vi "GDSString_CapsAndRemoveSpaces.vi"(10 "String":string) -> (2 "concatenated string":string)   [LabVIEW 2020]
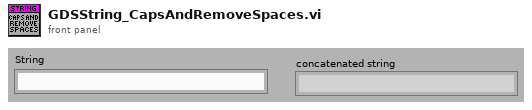
[diagram p1: front panel]
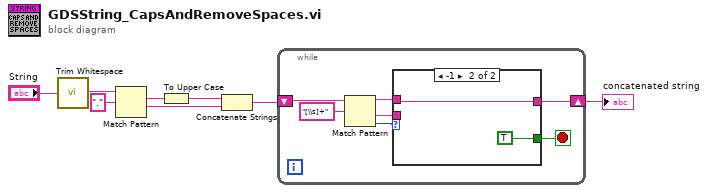
[diagram p0: block diagram]
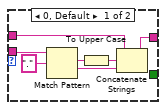
[diagram p2: hidden frame]
diagram:
  n1 = call <vilib>:"Trim Whitespace.vi"("string"="String") -> ("trimmed string"=w7:string)  [unwired: 1 in]
  n2 = Match Pattern(string=w7, regular expression=".") -> (match substring=w5:string, after substring=w3:string)  [unwired: 1 in, 2 out]
  n3 = To Upper Case(1:w5) -> (0:w4:string)
  n4 = Concatenate Strings(w4, w3) -> (w2:string)
  n5 = while {
    shift-right: [w10] -> w1
    shift-left: w2 -> [w15]
    stop <- w9 stop-if-true
    n6 = Match Pattern(string=w15, regular expression="[\\s]+") -> (before substring=w12:string, after substring=w11:string, offset past match=w13:i32)  [unwired: 1 in, 1 out]
    n7 = case shown="-1" w13 {
      tunnel: w12 -> [w17 w24]
      tunnel: w11 -> [w21 _]
      tunnel: [w16 w24] -> w10
      tunnel: [_ TRUE] -> w9
      frame 0, Default {
        n8 = Match Pattern(string=w21, regular expression=".") -> (match substring=w20:string, after substring=w18:string)  [unwired: 1 in, 2 out]
        n9 = To Upper Case(1:w20) -> (0:w19:string)
        n10 = Concatenate Strings(w17, w19, w18) -> (w16:string)
      }
      frame -1 {
      }
    }
  }
  "concatenated string" <- w1
